vi "tmp.vi"() -> ()   [LabVIEW 2015]
panel:
  in  "VgCluster":T1={"V1 (V)"=1.0, "Sweep rate, V/min"=1.0, "Time btw \npoints, sec"=1.0, "points at each Vg"=1, "Compliance, mkA"=0.05, "V2 (V)"=1.0, "No-record rate, V/min"=1.0, "Full sweep?"=TRUE} {"No-record rate, V/min" min=0.0 max=1.0 step=0.01 format="%_4f"; "V2 (V)" min=-4.0 max=4.0 step=0.1 format="%.1f"; "Compliance, mkA" min=0.0 max=1.0 step=0.01 format="%.3f"; "Time btw \npoints, sec" format="%.2f"; "Sweep rate, V/min" min=0.0 max=1.0 step=0.01 format="%_4f"; "V1 (V)" min=-4.0 max=4.0 step=0.1 format="%.1f"}
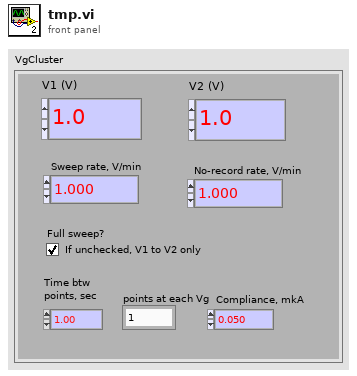
[diagram p1: front panel]
types:
  T1 = cluster{"V1 (V)":dbl, "Sweep rate, V/min":dbl, "Time btw \npoints, sec":dbl, "points at each Vg":i32, "Compliance, mkA":dbl, "V2 (V)":dbl, "No-record rate, V/min":dbl, "Full sweep?":bool}
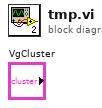
[diagram p0: block diagram]
diagram:
